vi "MotorShutDown.vi"(8 "error in (no error)":errorcluster caption="错误输入") -> (0 "error out":errorcluster caption="错误输出")   [LabVIEW 2018]
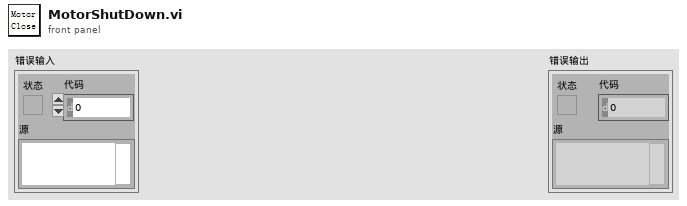
[diagram p1: front panel]
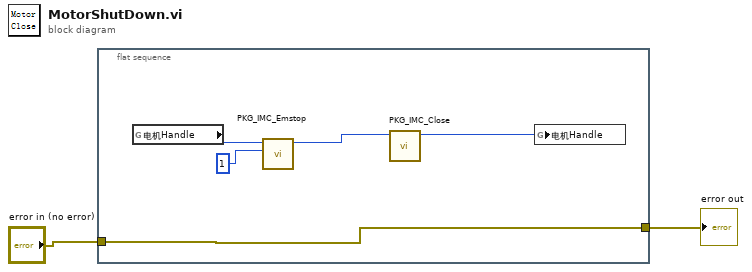
[diagram p0: block diagram]
diagram:
  n1 = flat-sequence {
    tunnel: "error in (no error)" -> [w3]
    tunnel: [w3] -> w1
    frame #0 {
      n2 = global read "参数.vi" "电机Handle"() -> (w5:u32)
      n3 = call "PKG_IMC_Emstop.vi"("isStop"=1, "Handle"=w5) -> ("Handle out"=w7:u32)  [unwired: 8 in, 1 out]
      n4 = call "PKG_IMC_Close.vi"("Handle"=w7) -> ("Handle out"=w4:u32)  [unwired: 9 in, 1 out]
      n5 = global write "参数.vi" "电机Handle"(w4) -> ()
    }
  }
  "error out" <- w1
